vi "detector_acquire_generic_data.vi"(8 "error in (no error)":errorcluster, 11 "hydraharp in":refnum<class "hydraharp.lvclass">) -> (0 "error out":errorcluster, 2 "image_data":T1, 3 "hydraharp out":refnum<class "hydraharp.lvclass">)   [LabVIEW 2015, in "hydraharp.lvclass"]
uses:
  hydraharp.lvclass
  Experiment/experiment_panel/2d_scan/detector_data_tdef.ctl
  hydraharp.lvclass/hydraharp.ctl
  <vilib>/Analysis/baseanly.llb/Mean (DBL).vi
  <vilib>/Analysis/NI_AALBase.lvlib
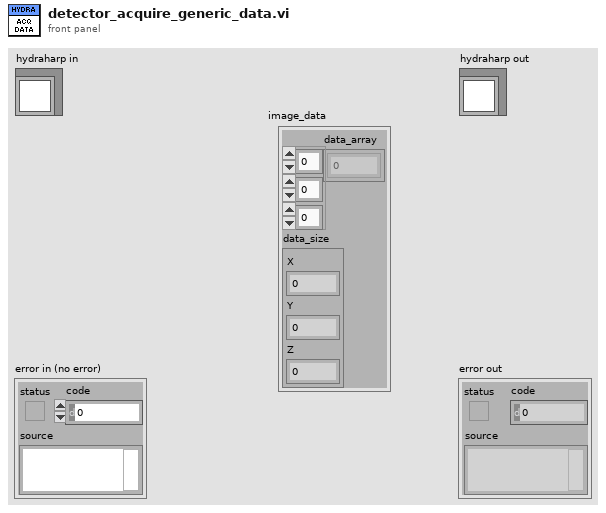
[diagram p1: front panel]
types:
  T1 = typedef "detector_data_tdef.ctl" = cluster{"data_array":dbl[][][], "data_size":cluster{"X":i32, "Y":i32, "Z":i32}}
  T2 = typedef "hydraharp_count_rates.ctl" = cluster{"channel_rates":i32[], "sync_rate":i32}
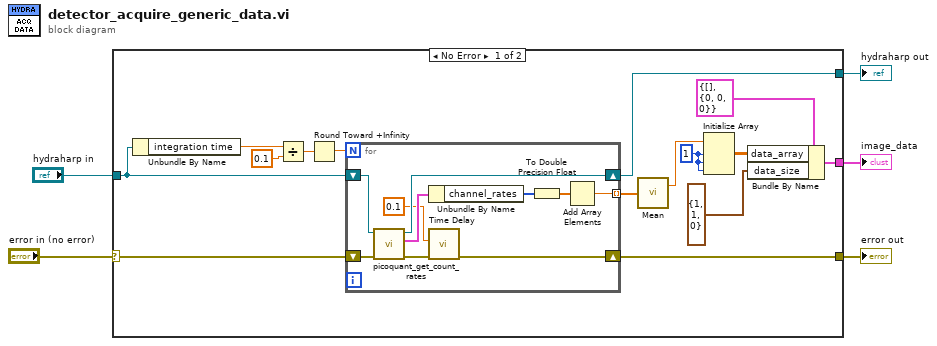
[diagram p0: block diagram]
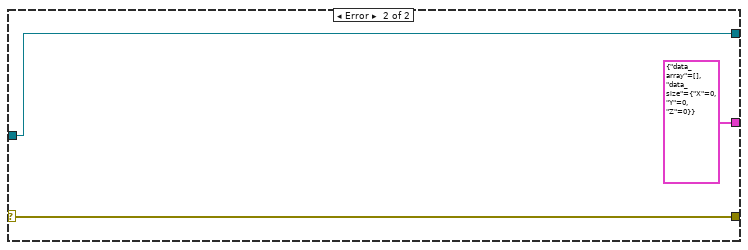
[diagram p2: hidden frame]
diagram:
  n1 = case shown="No Error" "error in (no error)" {
    selector: "error in (no error)" -> [w15 w31]
    tunnel: "hydraharp in" -> [w16 w33]
    tunnel: [w14 w33] -> w3
    tunnel: [w13 w31] -> w2
    tunnel: [w7 T1 {"data_array"=[], "data_size"={"X"=0, "Y"=0, "Z"=0}} ("image_data")] -> w1
    frame No Error {
      w11 = 1 ("dimension size")
      n2 = Unbundle By Name(w16) -> ("integration time"=w20:dbl)
      n3 = Divide(x=w20, y=0.1) -> (x/y=w18:dbl)
      n4 = Round Toward +Infinity(x=w18) -> (ceil(x): smallest int >= x=w17:dbl)
      n5 = for {
        N: w17 -> [_]
        shift-right: [w27] -> w14
        shift-left: w16 -> [w28]
        shift-right: [w23] -> w13
        shift-left: w15 -> [w26]
        tunnel: [w21] -> w12 mode=indexing
        n6 = call-dynamic "picoquant_get_count_rates.vi"("error in (no error)"=w26, "hydraharp in"=w28) -> ("error out"=w24:errorcluster, "count_rates"=w30:T2, "hydraharp out"=w27:refnum<class "hydraharp.lvclass">)  [unwired: 7 in]
        n7 = Unbundle By Name(w30) -> ("channel_rates"=w29:i32[])
        n8 = call "Time Delay"("error in (no error)"=w24, "Delay Time (s)"=0.1) -> ("error out"=w23:errorcluster)  [unwired: 9 in]
        n9 = To Double Precision Float(number=w29) -> (double precision float=w22:dbl[])
        n10 = Add Array Elements(numeric array=w22) -> (sum=w21:dbl)
      }
      n11 = call-poly <vilib>:"Mean.vi"("X"=w12) -> ("mean"=w10:dbl)  [unwired: 1 out]
      n12 = Initialize Array(w10, w11, w11, w11) -> (w8:dbl[][][])
      n13 = Bundle By Name(cluster=T1 {"data_array"=[], "data_size"={"X"=0, "Y"=0, "Z"=0}} ("image_data"), "data_array"=w8, "data_size"=cluster{"X":i32, "Y":i32, "Z":i32} {"X"=1, "Y"=1, "Z"=0}) -> (w7:T1)
    }
    frame Error {
    }
  }
  "error out" <- w2
  "hydraharp out" <- w3
  "image_data" <- w1
